vi "PERFECT(spin).vi"() -> ()   [LabVIEW 2015]
uses:
  <vilib>/NXT/Block Support/NXT_InputPort.ctl
  <vilib>/NXT/Block Support/NXT_OutputPort.ctl
  <vilib>/NXT/Dual Mode Library/Sensors/Sonar_cm.vi
  <vilib>/NXT/NXTIO Xnodes/NXTIONodeSubVIs/NXTMoveMotors.vi
  <vilib>/NXT/Dual Mode Library/Sensors/Light_On.vi
  <vilib>/NXT/Dual Mode Library/Sensors/Touch_Pressed.vi
  <vilib>/NXT/Dual Mode Library/Waits/Wait_Num.vi
  <vilib>/NXT/Subs/LVHSConnector.ctl
  <vilib>/NXT/NXTIO Xnodes/AddressXNode/NXTIOAddress.xnode
  <vilib>/NXT/NXTIO Xnodes/NXTIOXNode/NXTIO.xnode
  <vilib>/NXT/LegoClasses/BrickReference/BrickReference.lvclass
panel:
  in  "흰선을 보면 후진":i8=75
  in  "Time (1 sec) 2":sgl=1.0
  in  "C바퀴만 3초 돈다":i8=75
  in  "B바퀴":i8=75
  in  "터치센서 누르면 5초 후진":i8=75
  in  "Time (1 sec)":sgl=1.0
  in  "stop":bool
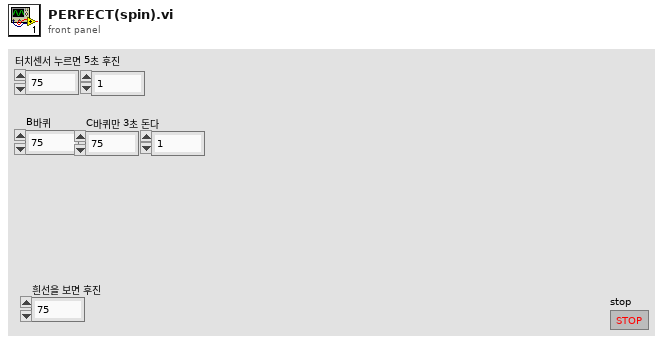
[diagram p1: front panel]
types:
  T1 = typedef "NXT_OutputPort.ctl" = u8
  T2 = typedef "NXT_InputPort.ctl" = u32
  T3 = typedef "LVHSConnector.ctl" = refnum<class "BrickReference.lvclass">
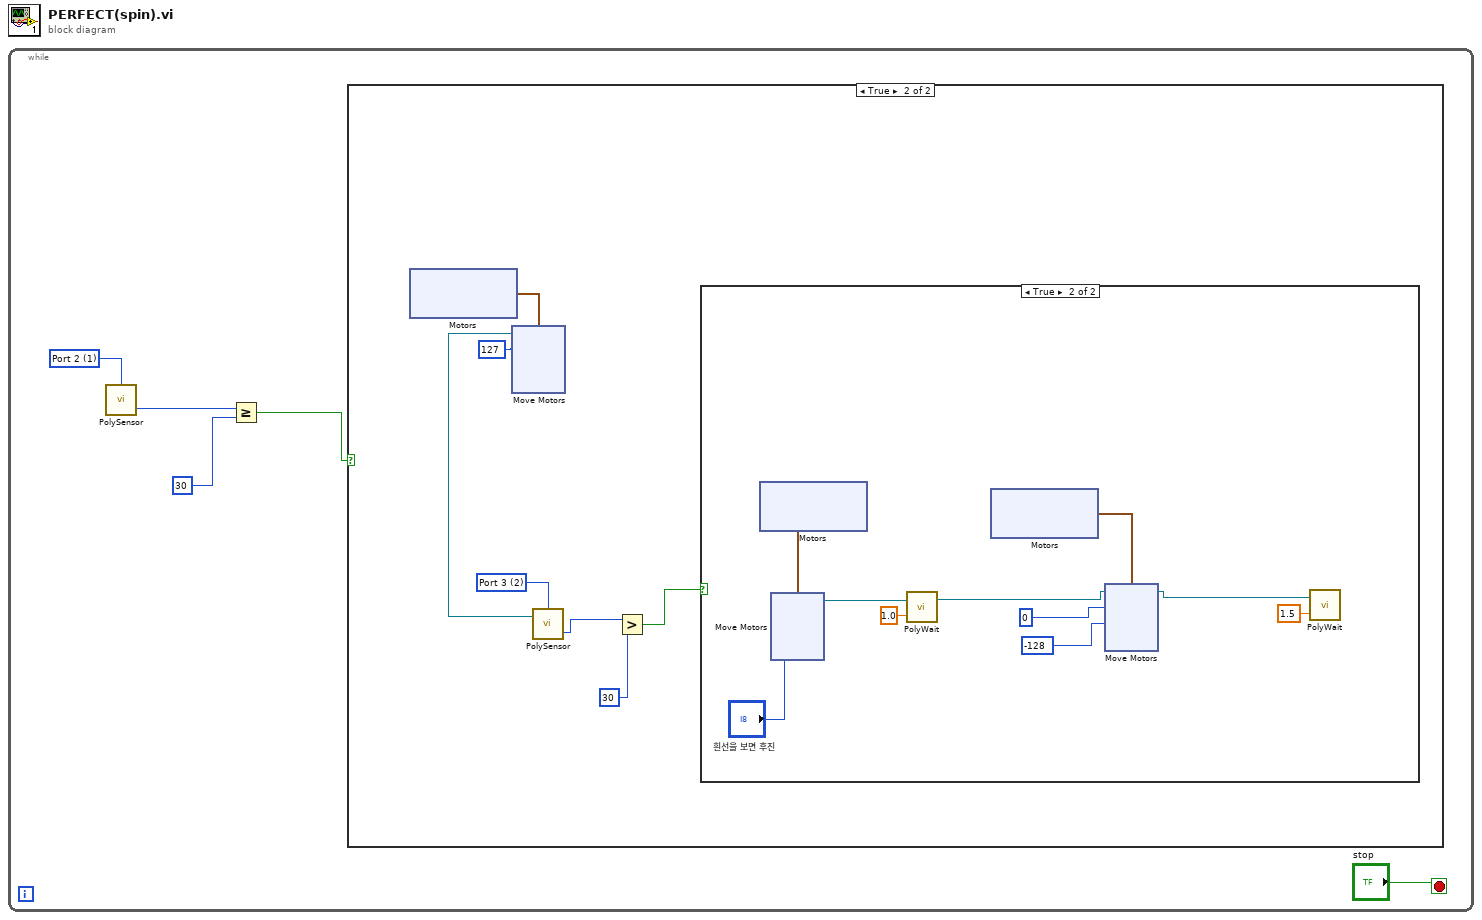
[diagram p0: block diagram]
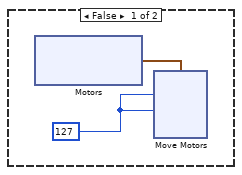
[diagram p2: hidden frame]
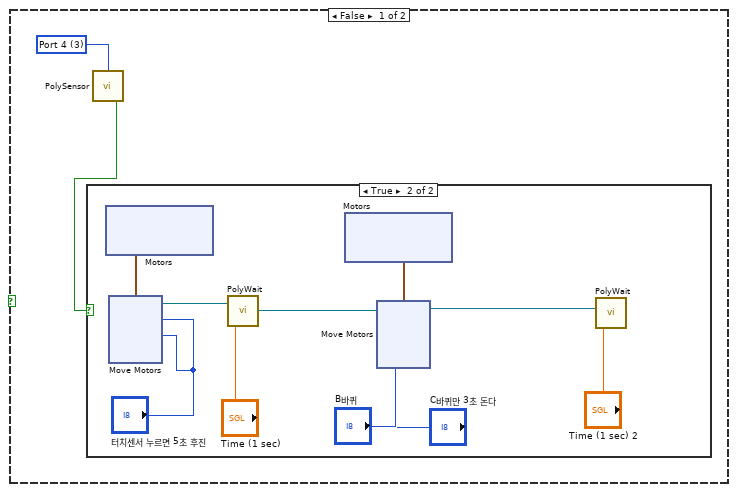
[diagram p3: hidden frame]
diagram:
  n1 = while {
    stop <- "stop" stop-if-true
    w4 = T2 1 items=["Port 1", "Port 2", "Port 3", "Port 4"] ("Port (Port 4)")
    n2 = call-poly <vilib>:"PolySensor.vi"("Port (Port 4)"=w4) -> ("Distance (cm)"=w2:i16)  [unwired: 2 in, 1 out]
    n3 = Greater Or Equal?(x=w2, y=i16 30) -> (x >= y?=w3:bool)
    n4 = case shown="True" w3 {
      frame False {
        w6 = i8 127 ("Power/Speed 1")
        n5 = xnode "Motors"() -> ("Motor"=w7:cluster{"Port":T1, "Port":T1})
        n6 = xnode "Move Motors"("Power/Speed 2"=w6, "Power/Speed 1"=w6, "Motors"=w7) -> ()  [unwired: 1 in, 1 out]
      }
      frame True {
        w17 = i8 127 ("Power/Speed 1")
        w22 = T2 2 items=["Port 1", "Port 2", "Port 3", "Port 4"] ("Port (Port 3)")
        n7 = xnode "Motors"() -> ("Motor"=w23:cluster{"Port":T1, "Port":T1})
        n8 = xnode "Move Motors"("Power/Speed 2"=w17, "Power/Speed 1"=w17, "Motors"=w23) -> ("NXT/EV3"=w18:T3)  [unwired: 1 in]
        n9 = call-poly <vilib>:"PolySensor.vi"("NXT/EV3"=w18, "Port (Port 3)"=w22) -> ("Scaled Value"=w20:i16)  [unwired: 1 in, 1 out]
        n10 = Greater?(x=w20, y=i16 30) -> (0:w21:bool)
        n11 = case shown="True" w21 {
          frame False {
            w34 = T2 3 items=["Port 1", "Port 2", "Port 3", "Port 4"] ("Port (Port 1)")
            n12 = call-poly <vilib>:"PolySensor.vi"("Port (Port 1)"=w34) -> ("Yes / No"=w33:bool)  [unwired: 2 in, 1 out]
            n13 = case shown="True" w33 {
              frame False {
              }
              frame True {
                n14 = xnode "Motors"() -> ("Motor"=w44:cluster{"Port":T1, "Port":T1})
                n15 = xnode "Move Motors"("Power/Speed 2"="터치센서 누르면 5초 후진", "Power/Speed 1"="터치센서 누르면 5초 후진", "Motors"=w44) -> ("NXT/EV3"=w38:T3)  [unwired: 1 in]
                n16 = call-poly <vilib>:"PolyWait.vi"("Time (1 sec)"="Time (1 sec)", "NXT/EV3"=w38) -> ("NXT/EV3"=w37:T3)  [unwired: 2 in]
                n17 = xnode "Motors"() -> ("Motor"=w43:cluster{"Port":T1, "Port":T1})
                n18 = xnode "Move Motors"("Power/Speed 2"="C바퀴만 3초 돈다", "Power/Speed 1"="B바퀴", "Motors"=w43, "NXT/EV3"=w37) -> ("NXT/EV3"=w36:T3)
                n19 = call-poly <vilib>:"PolyWait.vi"("Time (1 sec)"="Time (1 sec) 2", "NXT/EV3"=w36) -> ()  [unwired: 2 in, 1 out]
              }
            }
          }
          frame True {
            n20 = xnode "Motors"() -> ("Motor"=w64:cluster{"Port":T1, "Port":T1})
            n21 = xnode "Move Motors"("Power/Speed 2"="흰선을 보면 후진", "Power/Speed 1"="흰선을 보면 후진", "Motors"=w64) -> ("NXT/EV3"=w66:T3)  [unwired: 1 in]
            n22 = call-poly <vilib>:"PolyWait.vi"("Time (1 sec)"=sgl 1.0, "NXT/EV3"=w66) -> ("NXT/EV3"=w65:T3)  [unwired: 2 in]
            n23 = xnode "Motors"() -> ("Motor"=w72:cluster{"Port":T1, "Port":T1})
            n24 = xnode "Move Motors"("Power/Speed 2"=i8 -128, "Power/Speed 1"=i8 0, "Motors"=w72, "NXT/EV3"=w65) -> ("NXT/EV3"=w71:T3)
            n25 = call-poly <vilib>:"PolyWait.vi"("Time (1 sec)"=sgl 1.5, "NXT/EV3"=w71) -> ()  [unwired: 2 in, 1 out]
          }
        }
      }
    }
  }
